vi "angletostep.vi"(1 "Angle":i16) -> (0 "Step":i16)   [LabVIEW 2012]
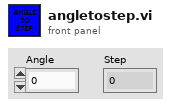
[diagram p1: front panel]
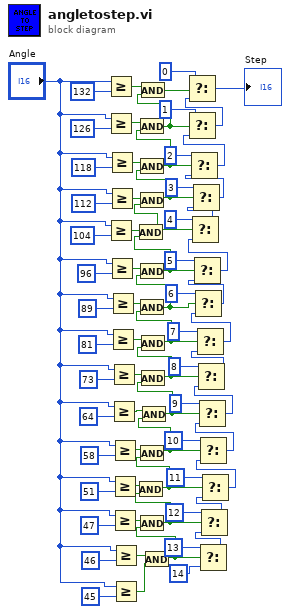
[diagram p0: block diagram]
diagram:
  n1 = Greater Or Equal?(x="Angle", y=i16 132) -> (x >= y?=w58:bool)
  n2 = Greater Or Equal?(x="Angle", y=i16 126) -> (x >= y?=w57:bool)
  n3 = Greater Or Equal?(x="Angle", y=i16 104) -> (x >= y?=w8:bool)
  n4 = Greater Or Equal?(x="Angle", y=i16 118) -> (x >= y?=w56:bool)
  n5 = Greater Or Equal?(x="Angle", y=i16 112) -> (x >= y?=w55:bool)
  n6 = Greater Or Equal?(x="Angle", y=i16 96) -> (x >= y?=w54:bool)
  n7 = Greater Or Equal?(x="Angle", y=i16 89) -> (x >= y?=w53:bool)
  n8 = Greater Or Equal?(x="Angle", y=i16 81) -> (x >= y?=w52:bool)
  n9 = Greater Or Equal?(x="Angle", y=i16 73) -> (x >= y?=w51:bool)
  n10 = Greater Or Equal?(x="Angle", y=i16 64) -> (x >= y?=w50:bool)
  n11 = Greater Or Equal?(x="Angle", y=i16 58) -> (x >= y?=w49:bool)
  n12 = Greater Or Equal?(x="Angle", y=i16 51) -> (x >= y?=w48:bool)
  n13 = Greater Or Equal?(x="Angle", y=i16 47) -> (x >= y?=w47:bool)
  n14 = Greater Or Equal?(x="Angle", y=i16 46) -> (x >= y?=w60:bool)
  n15 = Greater Or Equal?(x="Angle", y=i16 45) -> (x >= y?=w59:bool)
  n16 = And(x=w60, y=w59) -> (x .and. y?=w35:bool)
  n17 = And(x=w47, y=w35) -> (x .and. y?=w36:bool)
  n18 = And(x=w48, y=w36) -> (x .and. y?=w37:bool)
  n19 = And(x=w49, y=w37) -> (x .and. y?=w38:bool)
  n20 = And(x=w50, y=w38) -> (x .and. y?=w39:bool)
  n21 = And(x=w51, y=w39) -> (x .and. y?=w40:bool)
  n22 = And(x=w52, y=w40) -> (x .and. y?=w41:bool)
  n23 = And(x=w53, y=w41) -> (x .and. y?=w42:bool)
  n24 = And(x=w54, y=w42) -> (x .and. y?=w5:bool)
  n25 = And(x=w8, y=w5) -> (x .and. y?=w4:bool)
  n26 = And(x=w55, y=w4) -> (x .and. y?=w43:bool)
  n27 = And(x=w56, y=w43) -> (x .and. y?=w44:bool)
  n28 = And(x=w57, y=w44) -> (x .and. y?=w45:bool)
  n29 = And(x=w58, y=w45) -> (x .and. y?=w46:bool)
  n30 = Select(t=i16 13, s=w35, f=i16 14) -> (s? t:f=w26:i16)
  n31 = Select(t=i16 12, s=w36, f=w26) -> (s? t:f=w25:i16)
  n32 = Select(t=i16 11, s=w37, f=w25) -> (s? t:f=w24:i16)
  n33 = Select(t=i16 10, s=w38, f=w24) -> (s? t:f=w23:i16)
  n34 = Select(t=i16 9, s=w39, f=w23) -> (s? t:f=w22:i16)
  n35 = Select(t=i16 8, s=w40, f=w22) -> (s? t:f=w27:i16)
  n36 = Select(t=i16 7, s=w41, f=w27) -> (s? t:f=w28:i16)
  n37 = Select(t=i16 6, s=w42, f=w28) -> (s? t:f=w29:i16)
  n38 = Select(t=i16 5, s=w5, f=w29) -> (s? t:f=w3:i16)
  n39 = Select(t=i16 4, s=w4, f=w3) -> (s? t:f=w2:i16)
  n40 = Select(t=i16 3, s=w43, f=w2) -> (s? t:f=w30:i16)
  n41 = Select(t=i16 2, s=w44, f=w30) -> (s? t:f=w31:i16)
  n42 = Select(t=i16 1, s=w45, f=w31) -> (s? t:f=w32:i16)
  n43 = Select(t=i16 0, s=w46, f=w32) -> (s? t:f=→"Step":i16)
